vi "_f_BronkhorstModule.vi"(5 "Enable(T)":bool=TRUE, 6 "Delay":dbl=0.05, 7 "Command":T2, 8 "error in (no error)":errorcluster, 9 "Value":dbl, 10 "Nodo":u8=3, 11 "VISA resource name":refnum<visa-resource-name>="COM1") -> (0 "error out":errorcluster, 1 "Reading":T3, 2 "Result":string, 3 "Value":string)   [LabVIEW 2013]
uses:
  _f_BronkhorstModuleControl.ctl
  SerialComm/_f_SerialComm_Hardware_Module Control.ctl
panel:
  out "commandType":T1(ring)
  in  "InitComms":bool
  out "ReadString":string
  out "SendString":string
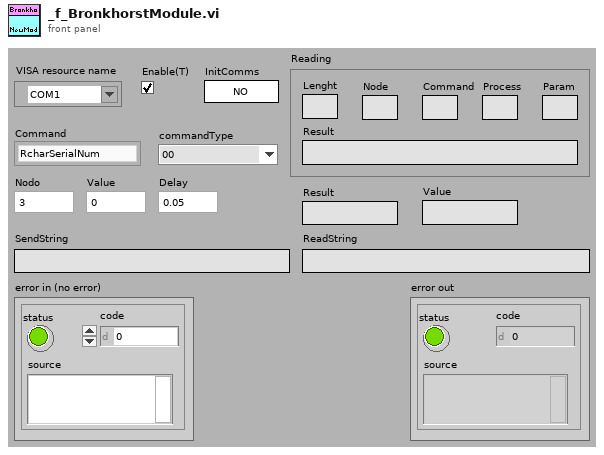
[diagram p1: front panel]
types:
  T1 = enum16{"00", "01", "02", "03", "04", "05", "06", "07", "08", "09"}
  T2 = typedef "_f_BronkhorstModuleControl.ctl" = enum16{"RcharSerialNum", "RcharIdnString", "WuintFluidNum", "RuintFluidNum", "RcharFluidName", "RuintSensorType", "RfloatCap0", "RfloatCap100", "RcharCapUnitStr", "W%Setpoint", "R%Setpoint", "R%Measure", "WfloatSetpoint", "RfloatSetpoint", "RfloatMeasure ", "RfloatDensity", "WuintControlMode", "WcharRESET", "RfloatCounter", "RcharCounterUnit", "WfloatCounterLimit", "RfloatCounterLimit", "WcharCounterMode", "RcharCounterMode", "WcharCounterSPMode", "RcharCounterSPMode", "WcharCounterNewSP", "RcharCounterNewSP"}
  T3 = cluster{"Lenght":string, "Node":string, "Process":string, "Param":string, "Command":string, "Result":string}
  T4 = typedef "_f_SerialComm_Hardware_Module Control.ctl" = enum16{"Initialize", "Write", "Bytes?", "Read", "Shutdown"}
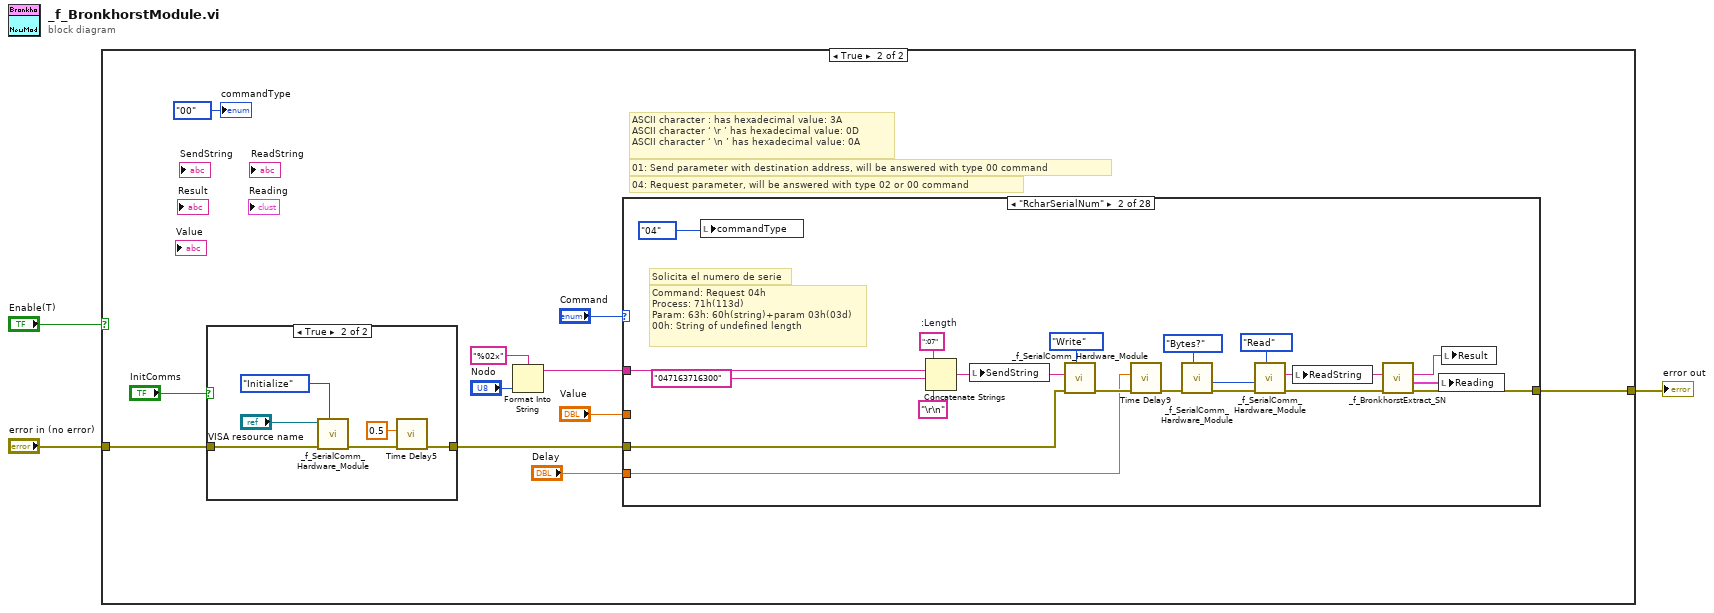
[diagram p0: block diagram]
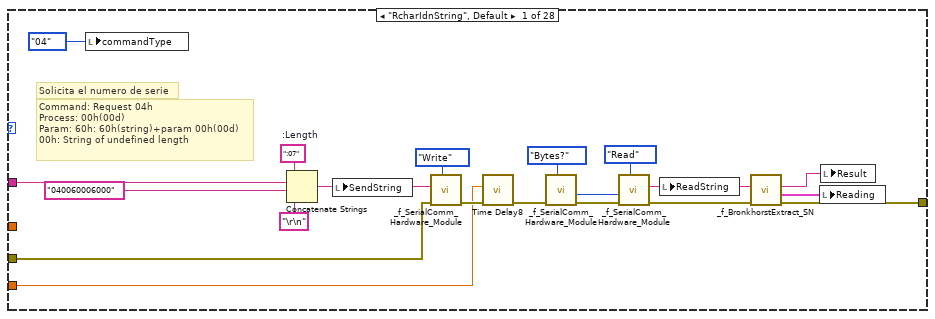
[diagram p4: hidden frame]
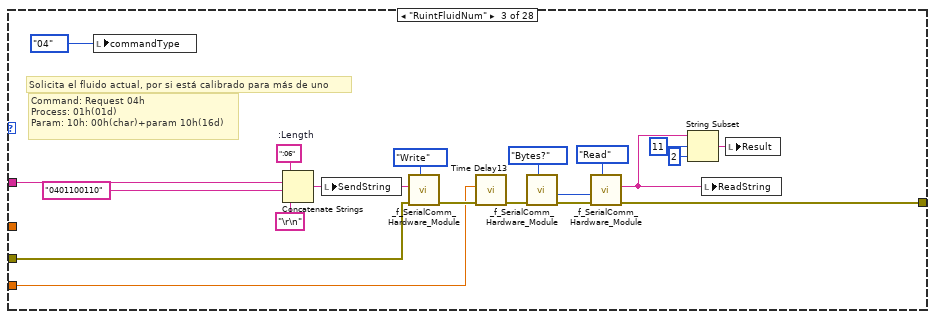
[diagram p5: hidden frame]
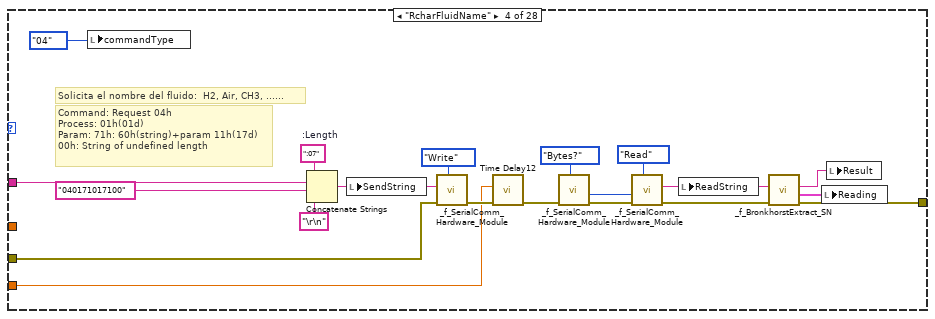
[diagram p6: hidden frame]
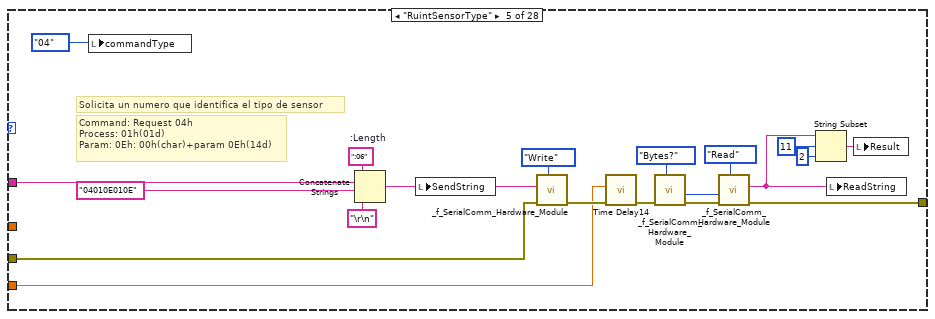
[diagram p7: hidden frame]
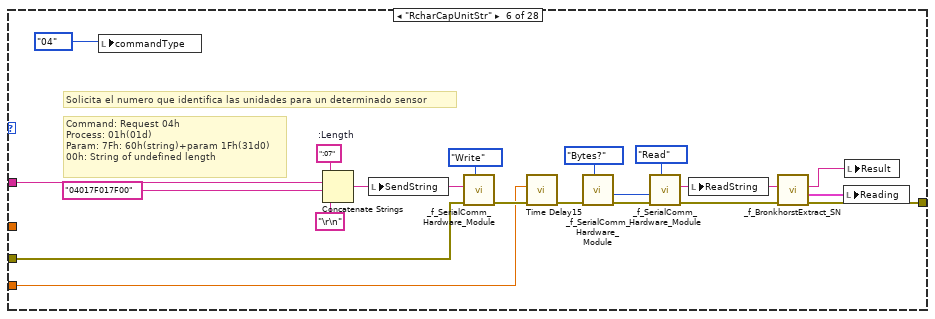
[diagram p8: hidden frame]
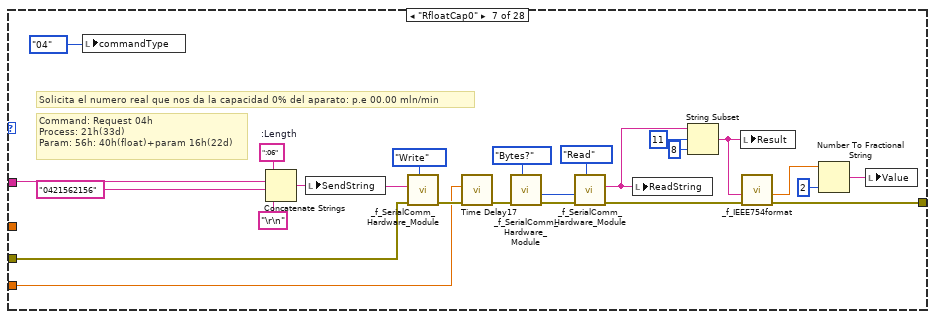
[diagram p9: hidden frame]
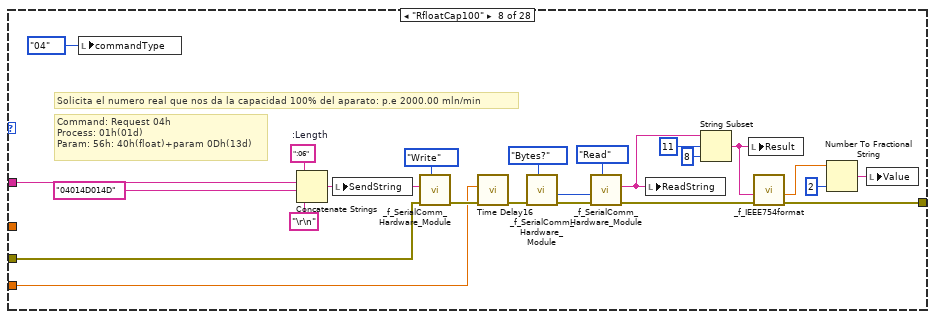
[diagram p10: hidden frame]
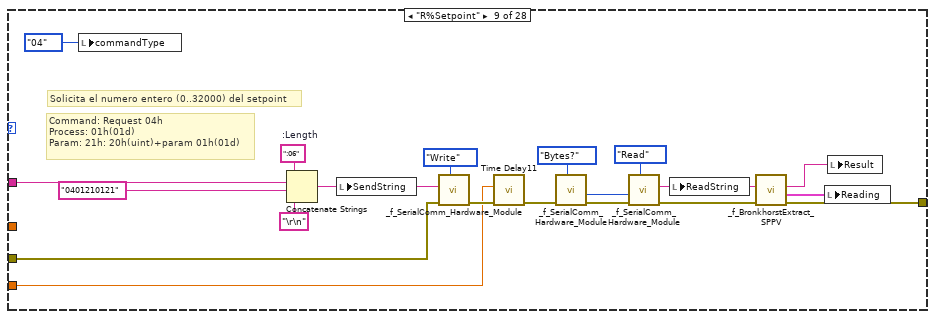
[diagram p11: hidden frame]
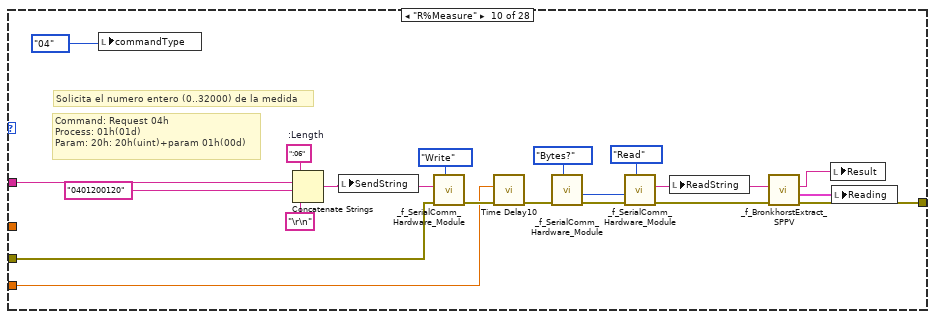
[diagram p12: hidden frame]
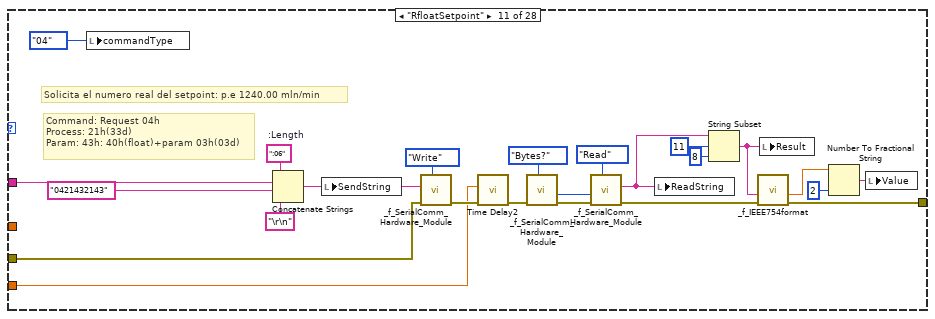
[diagram p13: hidden frame]
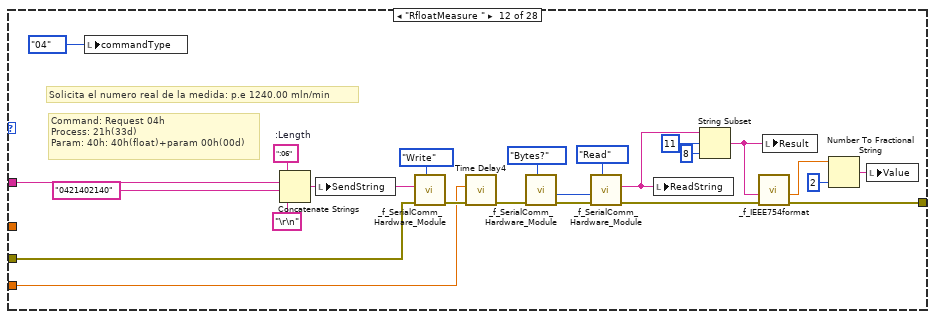
[diagram p14: hidden frame]
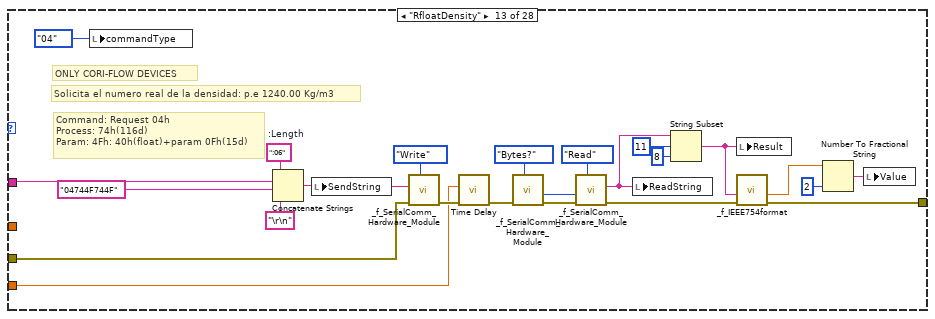
[diagram p15: hidden frame]
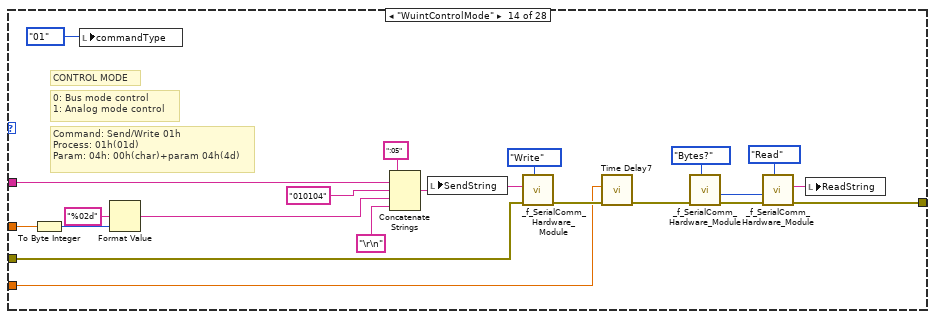
[diagram p16: hidden frame]
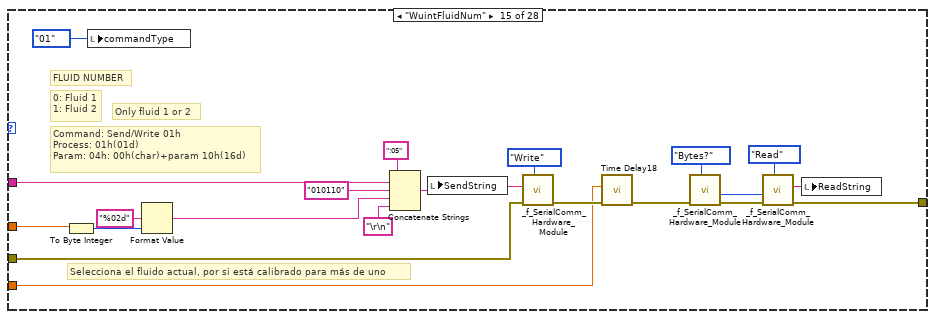
[diagram p17: hidden frame]
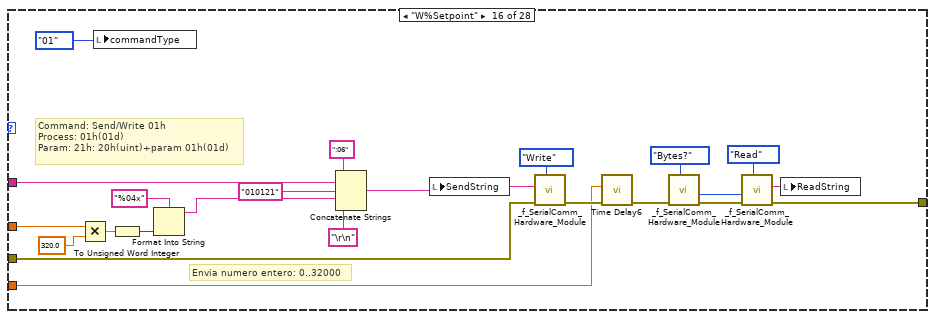
[diagram p18: hidden frame]
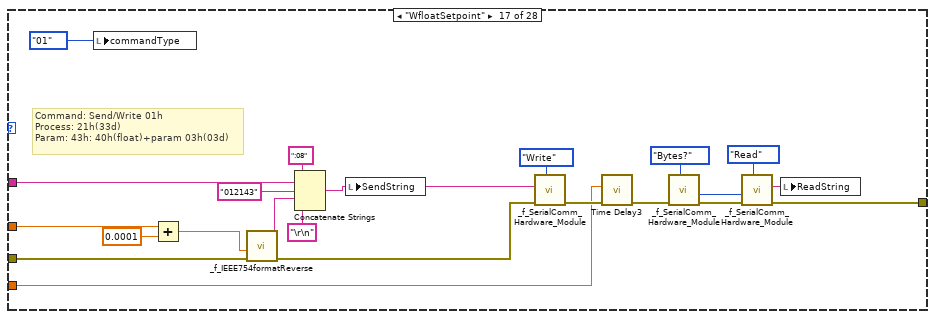
[diagram p19: hidden frame]
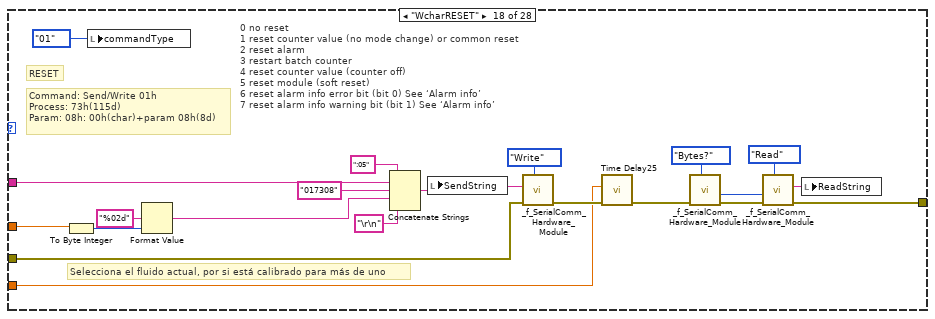
[diagram p20: hidden frame]
diagram:
  n1 = case shown="True" "Enable(T)" {
    tunnel: "error in (no error)" -> [w4 w14]
    tunnel: [w4 w5] -> w2
    frame False {
    }
    frame True {
      # "ASCII character : has hexadecimal value: 3A\nASCII character ‘ \\r ’ has hexadecimal value: 0D\nASCII character ‘ \\n ’ has hexadecimal value: 0A"
      # "04: Request parameter, will be answered with type 02 or 00 command"
      # "01: Send parameter with destination address, will be answered with type 00 command"
      n2 = case shown="True" "InitComms" {
        tunnel: w14 -> [w16 w21]
        tunnel: [w16 w18] -> w7
        frame False {
        }
        frame True {
          n3 = call "_f_SerialComm_Hardware_Module.vi"("Command"=_f_SerialComm_Hardware_Module_Control."Initialize", "error in (no error)"=w21, "VISA resource name"="VISA resource name") -> ("error out"=w19:errorcluster)  [unwired: 6 in, 2 out]
          n4 = call "Time Delay5"("error in (no error)"=w19, "Delay Time (s)"=0.5) -> ("error out"=w18:errorcluster)  [unwired: 9 in]
        }
      }
      n5 = Format Into String(format string="%02x", "Nodo") -> (resulting string=w10:string)  [unwired: 2 in, 1 out]
      n6 = case shown="\"RcharSerialNum\"" "Command" {
        tunnel: w10 -> [w24 w61 w64 w84 w104 w130 w144 w169 w193 w212 w233 w266 w281 w322 w343 w366 w388 w409 w413 w442 w473 w477 w518 w521 w559 w562 w602 w606]
        tunnel: w7 -> [w41 w59 w81 w101 w121 w141 w165 w189 w209 w229 w253 w277 w301 w320 w341 w363 w373 w407 w433 w453 w458 w497 w516 w538 w557 w579 w599 w622]
        tunnel: [w33 w51 w72 w93 w112 w124 w152 w173 w201 w221 w240 w259 w288 w311 w332 w354 w377 w398 w420 w436 w462 w484 w507 w529 w548 w570 w590 w614] -> w5
        tunnel: "Value" -> [_ _ _ _ _ _ _ _ _ _ _ _ _ w306 w326 w348 w374 w392 _ _ w459 _ w502 _ w543 _ w584 _]
        tunnel: "Delay" -> [w29 w46 w69 w89 w109 w134 w155 w179 w197 w217 w243 w270 w291 w310 w331 w346 w375 w397 w423 w446 w460 w487 w506 w526 w547 w567 w582 w610]
        frame "RcharIdnString", Default {
          w28 = ":07"  # :Length
          # "Command: Request 04h\nProcess: 00h(00d)\nParam: 60h: 60h(string)+param 00h(00d)\n00h: String of undefined length"
          # "Solicita el numero de serie"
          n7 = local write "commandType"(T1."04" ("commandType")) -> ()
          n8 = Concatenate Strings(w28, w24, "040060006000" ("string"), "\r\n" ("string")) -> (w25:string)
          n9 = local write "SendString"(w25) -> ()
          n10 = call "_f_SerialComm_Hardware_Module.vi"("Command"=_f_SerialComm_Hardware_Module_Control."Write", "error in (no error)"=w41, "Write string"=w25) -> ("error out"=w38:errorcluster)  [unwired: 6 in, 2 out]
          n11 = call "Time Delay8"("error in (no error)"=w38, "Delay Time (s)"=w29) -> ("error out"=w37:errorcluster)  [unwired: 9 in]
          n12 = call "_f_SerialComm_Hardware_Module.vi"("Command"=_f_SerialComm_Hardware_Module_Control."Bytes?", "error in (no error)"=w37) -> ("error out"=w36:errorcluster, "Bytes?"=w35:u32)  [unwired: 7 in, 1 out]
          n13 = call "_f_SerialComm_Hardware_Module.vi"("Command"=_f_SerialComm_Hardware_Module_Control."Read", "error in (no error)"=w36, "Bytes to read"=w35) -> ("error out"=w34:errorcluster, "Read string"=w32:string)  [unwired: 6 in, 1 out]
          n14 = local write "ReadString"(w32) -> ()
          n15 = call "_f_BronkhorstExtract_SN.vi"("error in (no error)"=w34, "Read String"=w32) -> ("error out"=w33:errorcluster, "Reading"=w31:T3, "Result"=w30:string)  [unwired: 7 in]
          n16 = local write "Reading"(w31) -> ()
          n17 = local write "Result"(w30) -> ()
        }
        frame "RcharSerialNum" {
          w62 = ":07"  # :Length
          # "Command: Request 04h\nProcess: 71h(113d)\nParam: 63h: 60h(string)+param 03h(03d)\n00h: String of undefined length"
          # "Solicita el numero de serie"
          n18 = local write "commandType"(T1."04" ("commandType")) -> ()
          n19 = Concatenate Strings(w62, w61, "047163716300" ("string"), "\r\n" ("string")) -> (w50:string)
          n20 = local write "SendString"(w50) -> ()
          n21 = call "_f_SerialComm_Hardware_Module.vi"("Command"=_f_SerialComm_Hardware_Module_Control."Write", "error in (no error)"=w59, "Write string"=w50) -> ("error out"=w56:errorcluster)  [unwired: 6 in, 2 out]
          n22 = call "Time Delay9"("error in (no error)"=w56, "Delay Time (s)"=w46) -> ("error out"=w55:errorcluster)  [unwired: 9 in]
          n23 = call "_f_SerialComm_Hardware_Module.vi"("Command"=_f_SerialComm_Hardware_Module_Control."Bytes?", "error in (no error)"=w55) -> ("error out"=w54:errorcluster, "Bytes?"=w53:u32)  [unwired: 7 in, 1 out]
          n24 = call "_f_SerialComm_Hardware_Module.vi"("Command"=_f_SerialComm_Hardware_Module_Control."Read", "error in (no error)"=w54, "Bytes to read"=w53) -> ("error out"=w52:errorcluster, "Read string"=w49:string)  [unwired: 6 in, 1 out]
          n25 = local write "ReadString"(w49) -> ()
          n26 = call "_f_BronkhorstExtract_SN.vi"("error in (no error)"=w52, "Read String"=w49) -> ("error out"=w51:errorcluster, "Reading"=w48:T3, "Result"=w47:string)  [unwired: 7 in]
          n27 = local write "Reading"(w48) -> ()
          n28 = local write "Result"(w47) -> ()
        }
        frame "RuintFluidNum" {
          w68 = ":06"  # :Length
          # "Command: Request 04h\nProcess: 01h(01d)\nParam: 10h: 00h(char)+param 10h(16d)"
          # "Solicita el fluido actual, por si está calibrado para más de uno"
          n29 = local write "commandType"(T1."04" ("commandType")) -> ()
          n30 = Concatenate Strings(w68, w64, "0401100110" ("string"), "\r\n" ("string")) -> (w65:string)
          n31 = local write "SendString"(w65) -> ()
          n32 = call "_f_SerialComm_Hardware_Module.vi"("Command"=_f_SerialComm_Hardware_Module_Control."Write", "error in (no error)"=w81, "Write string"=w65) -> ("error out"=w78:errorcluster)  [unwired: 6 in, 2 out]
          n33 = call "Time Delay13"("error in (no error)"=w78, "Delay Time (s)"=w69) -> ("error out"=w77:errorcluster)  [unwired: 9 in]
          n34 = call "_f_SerialComm_Hardware_Module.vi"("Command"=_f_SerialComm_Hardware_Module_Control."Bytes?", "error in (no error)"=w77) -> ("error out"=w76:errorcluster, "Bytes?"=w75:u32)  [unwired: 7 in, 1 out]
          n35 = call "_f_SerialComm_Hardware_Module.vi"("Command"=_f_SerialComm_Hardware_Module_Control."Read", "error in (no error)"=w76, "Bytes to read"=w75) -> ("error out"=w72:errorcluster, "Read string"=w73:string)  [unwired: 6 in, 1 out]
          n36 = String Subset(string=w73, offset (0)=11, length (rest)=2 ("length (rest)")) -> (substring=w70:string)
          n37 = local write "ReadString"(w73) -> ()
          n38 = local write "Result"(w70) -> ()
        }
        frame "RcharFluidName" {
          w88 = ":07"  # :Length
          # "Command: Request 04h\nProcess: 01h(01d)\nParam: 71h: 60h(string)+param 11h(17d)\n00h: String of undefined length"
          # "Solicita el nombre del fluido:  H2, Air, CH3, ......"
          n39 = local write "commandType"(T1."04" ("commandType")) -> ()
          n40 = Concatenate Strings(w88, w84, "040171017100" ("string"), "\r\n" ("string")) -> (w85:string)
          n41 = local write "SendString"(w85) -> ()
          n42 = call "_f_SerialComm_Hardware_Module.vi"("Command"=_f_SerialComm_Hardware_Module_Control."Write", "error in (no error)"=w101, "Write string"=w85) -> ("error out"=w98:errorcluster)  [unwired: 6 in, 2 out]
          n43 = call "Time Delay12"("error in (no error)"=w98, "Delay Time (s)"=w89) -> ("error out"=w97:errorcluster)  [unwired: 9 in]
          n44 = call "_f_SerialComm_Hardware_Module.vi"("Command"=_f_SerialComm_Hardware_Module_Control."Bytes?", "error in (no error)"=w97) -> ("error out"=w96:errorcluster, "Bytes?"=w95:u32)  [unwired: 7 in, 1 out]
          n45 = call "_f_SerialComm_Hardware_Module.vi"("Command"=_f_SerialComm_Hardware_Module_Control."Read", "error in (no error)"=w96, "Bytes to read"=w95) -> ("error out"=w94:errorcluster, "Read string"=w92:string)  [unwired: 6 in, 1 out]
          n46 = local write "ReadString"(w92) -> ()
          n47 = call "_f_BronkhorstExtract_SN.vi"("error in (no error)"=w94, "Read String"=w92) -> ("error out"=w93:errorcluster, "Reading"=w91:T3, "Result"=w90:string)  [unwired: 7 in]
          n48 = local write "Reading"(w91) -> ()
          n49 = local write "Result"(w90) -> ()
        }
        frame "RuintSensorType" {
          w108 = ":06"  # :Length
          # "Command: Request 04h\nProcess: 01h(01d)\nParam: 0Eh: 00h(char)+param 0Eh(14d)"
          # "Solicita un numero que identifica el tipo de sensor"
          n50 = local write "commandType"(T1."04" ("commandType")) -> ()
          n51 = Concatenate Strings(w108, w104, "04010E010E" ("string"), "\r\n" ("string")) -> (w105:string)
          n52 = local write "SendString"(w105) -> ()
          n53 = call "_f_SerialComm_Hardware_Module.vi"("Command"=_f_SerialComm_Hardware_Module_Control."Write", "error in (no error)"=w121, "Write string"=w105) -> ("error out"=w118:errorcluster)  [unwired: 6 in, 2 out]
          n54 = call "Time Delay14"("error in (no error)"=w118, "Delay Time (s)"=w109) -> ("error out"=w117:errorcluster)  [unwired: 9 in]
          n55 = call "_f_SerialComm_Hardware_Module.vi"("Command"=_f_SerialComm_Hardware_Module_Control."Bytes?", "error in (no error)"=w117) -> ("error out"=w116:errorcluster, "Bytes?"=w115:u32)  [unwired: 7 in, 1 out]
          n56 = call "_f_SerialComm_Hardware_Module.vi"("Command"=_f_SerialComm_Hardware_Module_Control."Read", "error in (no error)"=w116, "Bytes to read"=w115) -> ("error out"=w112:errorcluster, "Read string"=w113:string)  [unwired: 6 in, 1 out]
          n57 = String Subset(string=w113, offset (0)=11, length (rest)=2 ("length (rest)")) -> (substring=w110:string)
          n58 = local write "ReadString"(w113) -> ()
          n59 = local write "Result"(w110) -> ()
        }
        frame "RcharCapUnitStr" {
          w133 = ":07"  # :Length
          # "Command: Request 04h\nProcess: 01h(01d)\nParam: 7Fh: 60h(string)+param 1Fh(31d0)\n00h: String of undefined length"
          # "Solicita el numero que identifica las unidades para un determinado sensor"
          n60 = local write "commandType"(T1."04" ("commandType")) -> ()
          n61 = Concatenate Strings(w133, w130, "04017F017F00" ("string"), "\r\n" ("string")) -> (w129:string)
          n62 = local write "SendString"(w129) -> ()
          n63 = call "_f_SerialComm_Hardware_Module.vi"("Command"=_f_SerialComm_Hardware_Module_Control."Write", "error in (no error)"=w141, "Write string"=w129) -> ("error out"=w138:errorcluster)  [unwired: 6 in, 2 out]
          n64 = call "Time Delay15"("error in (no error)"=w138, "Delay Time (s)"=w134) -> ("error out"=w137:errorcluster)  [unwired: 9 in]
          n65 = call "_f_SerialComm_Hardware_Module.vi"("Command"=_f_SerialComm_Hardware_Module_Control."Bytes?", "error in (no error)"=w137) -> ("error out"=w136:errorcluster, "Bytes?"=w135:u32)  [unwired: 7 in, 1 out]
          n66 = call "_f_SerialComm_Hardware_Module.vi"("Command"=_f_SerialComm_Hardware_Module_Control."Read", "error in (no error)"=w136, "Bytes to read"=w135) -> ("error out"=w125:errorcluster, "Read string"=w128:string)  [unwired: 6 in, 1 out]
          n67 = local write "ReadString"(w128) -> ()
          n68 = call "_f_BronkhorstExtract_SN.vi"("error in (no error)"=w125, "Read String"=w128) -> ("error out"=w124:errorcluster, "Reading"=w126:T3, "Result"=w127:string)  [unwired: 7 in]
          n69 = local write "Reading"(w126) -> ()
          n70 = local write "Result"(w127) -> ()
        }
        frame "RfloatCap0" {
          w148 = ":06"  # :Length
          # "Command: Request 04h\nProcess: 21h(33d)\nParam: 56h: 40h(float)+param 16h(22d)"
          # "Solicita el numero real que nos da la capacidad 0% del aparato: p.e 00.00 mln/min"
          n71 = local write "commandType"(T1."04" ("commandType")) -> ()
          n72 = Concatenate Strings(w148, w144, "0421562156" ("string"), "\r\n" ("string")) -> (w145:string)
          n73 = local write "SendString"(w145) -> ()
          n74 = call "_f_SerialComm_Hardware_Module.vi"("Command"=_f_SerialComm_Hardware_Module_Control."Write", "error in (no error)"=w165, "Write string"=w145) -> ("error out"=w162:errorcluster)  [unwired: 6 in, 2 out]
          n75 = call "Time Delay17"("error in (no error)"=w162, "Delay Time (s)"=w155) -> ("error out"=w161:errorcluster)  [unwired: 9 in]
          n76 = call "_f_SerialComm_Hardware_Module.vi"("Command"=_f_SerialComm_Hardware_Module_Control."Bytes?", "error in (no error)"=w161) -> ("error out"=w160:errorcluster, "Bytes?"=w159:u32)  [unwired: 7 in, 1 out]
          n77 = call "_f_SerialComm_Hardware_Module.vi"("Command"=_f_SerialComm_Hardware_Module_Control."Read", "error in (no error)"=w160, "Bytes to read"=w159) -> ("error out"=w153:errorcluster, "Read string"=w157:string)  [unwired: 6 in, 1 out]
          n78 = local write "ReadString"(w157) -> ()
          n79 = String Subset(string=w157, offset (0)=11, length (rest)=8 ("length (rest)")) -> (substring=w154:string)
          n80 = local write "Result"(w154) -> ()
          n81 = call "_f_IEEE754format.vi"("error in (no error)"=w153, "String"=w154) -> ("error out"=w152:errorcluster, "Number"=w149:sgl)  [unwired: 8 in]
          n82 = Number To Fractional String(number=w149, precision (6)=i16 2) -> (F-format string=w150:string)  [unwired: 2 in]
          n83 = local write "Value"(w150) -> ()
        }
        frame "RfloatCap100" {
          w172 = ":06"  # :Length
          # "Command: Request 04h\nProcess: 01h(01d)\nParam: 56h: 40h(float)+param 0Dh(13d)"
          # "Solicita el numero real que nos da la capacidad 100% del aparato: p.e 2000.00 mln/min"
          n84 = local write "commandType"(T1."04" ("commandType")) -> ()
          n85 = Concatenate Strings(w172, w169, "04014D014D" ("string"), "\r\n" ("string")) -> (w168:string)
          n86 = local write "SendString"(w168) -> ()
          n87 = call "_f_SerialComm_Hardware_Module.vi"("Command"=_f_SerialComm_Hardware_Module_Control."Write", "error in (no error)"=w189, "Write string"=w168) -> ("error out"=w186:errorcluster)  [unwired: 6 in, 2 out]
          n88 = call "Time Delay16"("error in (no error)"=w186, "Delay Time (s)"=w179) -> ("error out"=w185:errorcluster)  [unwired: 9 in]
          n89 = call "_f_SerialComm_Hardware_Module.vi"("Command"=_f_SerialComm_Hardware_Module_Control."Bytes?", "error in (no error)"=w185) -> ("error out"=w184:errorcluster, "Bytes?"=w183:u32)  [unwired: 7 in, 1 out]
          n90 = call "_f_SerialComm_Hardware_Module.vi"("Command"=_f_SerialComm_Hardware_Module_Control."Read", "error in (no error)"=w184, "Bytes to read"=w183) -> ("error out"=w174:errorcluster, "Read string"=w181:string)  [unwired: 6 in, 1 out]
          n91 = local write "ReadString"(w181) -> ()
          n92 = String Subset(string=w181, offset (0)=11, length (rest)=8 ("length (rest)")) -> (substring=w176:string)
          n93 = local write "Result"(w176) -> ()
          n94 = call "_f_IEEE754format.vi"("error in (no error)"=w174, "String"=w176) -> ("error out"=w173:errorcluster, "Number"=w175:sgl)  [unwired: 8 in]
          n95 = Number To Fractional String(number=w175, precision (6)=i16 2) -> (F-format string=w177:string)  [unwired: 2 in]
          n96 = local write "Value"(w177) -> ()
        }
        frame "R%Setpoint" {
          w196 = ":06"  # :Length
          # "Command: Request 04h\nProcess: 01h(01d)\nParam: 21h: 20h(uint)+param 01h(01d)"
          # "Solicita el numero entero (0..32000) del setpoint"
          n97 = local write "commandType"(T1."04" ("commandType")) -> ()
          n98 = Concatenate Strings(w196, w193, "0401210121" ("string"), "\r\n" ("string")) -> (w192:string)
          n99 = local write "SendString"(w192) -> ()
          n100 = call "_f_SerialComm_Hardware_Module.vi"("Command"=_f_SerialComm_Hardware_Module_Control."Write", "error in (no error)"=w209, "Write string"=w192) -> ("error out"=w206:errorcluster)  [unwired: 6 in, 2 out]
          n101 = call "Time Delay11"("error in (no error)"=w206, "Delay Time (s)"=w197) -> ("error out"=w205:errorcluster)  [unwired: 9 in]
          n102 = call "_f_SerialComm_Hardware_Module.vi"("Command"=_f_SerialComm_Hardware_Module_Control."Bytes?", "error in (no error)"=w205) -> ("error out"=w204:errorcluster, "Bytes?"=w203:u32)  [unwired: 7 in, 1 out]
          n103 = call "_f_SerialComm_Hardware_Module.vi"("Command"=_f_SerialComm_Hardware_Module_Control."Read", "error in (no error)"=w204, "Bytes to read"=w203) -> ("error out"=w202:errorcluster, "Read string"=w200:string)  [unwired: 6 in, 1 out]
          n104 = local write "ReadString"(w200) -> ()
          n105 = call "_f_BronkhorstExtract_SPPV.vi"("error in (no error)"=w202, "Read String"=w200) -> ("error out"=w201:errorcluster, "Reading"=w199:T3, "Setpoint"=w198:string)  [unwired: 7 in]
          n106 = local write "Reading"(w199) -> ()
          n107 = local write "Result"(w198) -> ()
        }
        frame "R%Measure" {
          w216 = ":06"  # :Length
          # "Command: Request 04h\nProcess: 01h(01d)\nParam: 20h: 20h(uint)+param 01h(00d)"
          # "Solicita el numero entero (0..32000) de la medida"
          n108 = local write "commandType"(T1."04" ("commandType")) -> ()
          n109 = Concatenate Strings(w216, w212, "0401200120" ("string"), "\r\n" ("string")) -> (w213:string)
          n110 = local write "SendString"(w213) -> ()
          n111 = call "_f_SerialComm_Hardware_Module.vi"("Command"=_f_SerialComm_Hardware_Module_Control."Write", "error in (no error)"=w229, "Write string"=w213) -> ("error out"=w226:errorcluster)  [unwired: 6 in, 2 out]
          n112 = call "Time Delay10"("error in (no error)"=w226, "Delay Time (s)"=w217) -> ("error out"=w225:errorcluster)  [unwired: 9 in]
          n113 = call "_f_SerialComm_Hardware_Module.vi"("Command"=_f_SerialComm_Hardware_Module_Control."Bytes?", "error in (no error)"=w225) -> ("error out"=w224:errorcluster, "Bytes?"=w223:u32)  [unwired: 7 in, 1 out]
          n114 = call "_f_SerialComm_Hardware_Module.vi"("Command"=_f_SerialComm_Hardware_Module_Control."Read", "error in (no error)"=w224, "Bytes to read"=w223) -> ("error out"=w222:errorcluster, "Read string"=w219:string)  [unwired: 6 in, 1 out]
          n115 = local write "ReadString"(w219) -> ()
          n116 = call "_f_BronkhorstExtract_SPPV.vi"("error in (no error)"=w222, "Read String"=w219) -> ("error out"=w221:errorcluster, "Reading"=w220:T3, "Setpoint"=w218:string)  [unwired: 7 in]
          n117 = local write "Result"(w218) -> ()
          n118 = local write "Reading"(w220) -> ()
        }
        frame "RfloatSetpoint" {
          w236 = ":06"  # :Length
          # "Command: Request 04h\nProcess: 21h(33d)\nParam: 43h: 40h(float)+param 03h(03d)"
          # "Solicita el numero real del setpoint: p.e 1240.00 mln/min"
          n119 = local write "commandType"(T1."04" ("commandType")) -> ()
          n120 = Concatenate Strings(w236, w233, "0421432143" ("string"), "\r\n" ("string")) -> (w232:string)
          n121 = local write "SendString"(w232) -> ()
          n122 = call "_f_SerialComm_Hardware_Module.vi"("Command"=_f_SerialComm_Hardware_Module_Control."Write", "error in (no error)"=w253, "Write string"=w232) -> ("error out"=w250:errorcluster)  [unwired: 6 in, 2 out]
          n123 = call "Time Delay2"("error in (no error)"=w250, "Delay Time (s)"=w243) -> ("error out"=w249:errorcluster)  [unwired: 9 in]
          n124 = call "_f_SerialComm_Hardware_Module.vi"("Command"=_f_SerialComm_Hardware_Module_Control."Bytes?", "error in (no error)"=w249) -> ("error out"=w248:errorcluster, "Bytes?"=w247:u32)  [unwired: 7 in, 1 out]
          n125 = call "_f_SerialComm_Hardware_Module.vi"("Command"=_f_SerialComm_Hardware_Module_Control."Read", "error in (no error)"=w248, "Bytes to read"=w247) -> ("error out"=w241:errorcluster, "Read string"=w245:string)  [unwired: 6 in, 1 out]
          n126 = local write "ReadString"(w245) -> ()
          n127 = String Subset(string=w245, offset (0)=11, length (rest)=8 ("length (rest)")) -> (substring=w242:string)
          n128 = call "_f_IEEE754format.vi"("error in (no error)"=w241, "String"=w242) -> ("error out"=w240:errorcluster, "Number"=w238:sgl)  [unwired: 8 in]
          n129 = local write "Result"(w242) -> ()
          n130 = Number To Fractional String(number=w238, precision (6)=i16 2) -> (F-format string=w237:string)  [unwired: 2 in]
          n131 = local write "Value"(w237) -> ()
        }
        frame "RfloatMeasure " {
          w269 = ":06"  # :Length
          # "Command: Request 04h\nProcess: 21h(33d)\nParam: 40h: 40h(float)+param 00h(00d)"
          # "Solicita el numero real de la medida: p.e 1240.00 mln/min"
          n132 = local write "commandType"(T1."04" ("commandType")) -> ()
          n133 = Concatenate Strings(w269, w266, "0421402140" ("string"), "\r\n" ("string")) -> (w265:string)
          n134 = local write "SendString"(w265) -> ()
          n135 = call "_f_SerialComm_Hardware_Module.vi"("Command"=_f_SerialComm_Hardware_Module_Control."Write", "error in (no error)"=w277, "Write string"=w265) -> ("error out"=w274:errorcluster)  [unwired: 6 in, 2 out]
          n136 = call "Time Delay4"("error in (no error)"=w274, "Delay Time (s)"=w270) -> ("error out"=w273:errorcluster)  [unwired: 9 in]
          n137 = call "_f_SerialComm_Hardware_Module.vi"("Command"=_f_SerialComm_Hardware_Module_Control."Bytes?", "error in (no error)"=w273) -> ("error out"=w272:errorcluster, "Bytes?"=w271:u32)  [unwired: 7 in, 1 out]
          n138 = call "_f_SerialComm_Hardware_Module.vi"("Command"=_f_SerialComm_Hardware_Module_Control."Read", "error in (no error)"=w272, "Bytes to read"=w271) -> ("error out"=w260:errorcluster, "Read string"=w258:string)  [unwired: 6 in, 1 out]
          n139 = local write "ReadString"(w258) -> ()
          n140 = String Subset(string=w258, offset (0)=11, length (rest)=8 ("length (rest)")) -> (substring=w257:string)
          n141 = call "_f_IEEE754format.vi"("error in (no error)"=w260, "String"=w257) -> ("error out"=w259:errorcluster, "Number"=w256:sgl)  [unwired: 8 in]
          n142 = local write "Result"(w257) -> ()
          n143 = Number To Fractional String(number=w256, precision (6)=i16 2) -> (F-format string=w261:string)  [unwired: 2 in]
          n144 = local write "Value"(w261) -> ()
        }
        frame "RfloatDensity" {
          w284 = ":06"  # :Length
          # "ONLY CORI-FLOW DEVICES"
          # "Command: Request 04h\nProcess: 74h(116d)\nParam: 4Fh: 40h(float)+param 0Fh(15d)"
          # "Solicita el numero real de la densidad: p.e 1240.00 Kg/m3"
          n145 = local write "commandType"(T1."04" ("commandType")) -> ()
          n146 = Concatenate Strings(w284, w281, "04744F744F" ("string"), "\r\n" ("string")) -> (w280:string)
          n147 = local write "SendString"(w280) -> ()
          n148 = call "_f_SerialComm_Hardware_Module.vi"("Command"=_f_SerialComm_Hardware_Module_Control."Write", "error in (no error)"=w301, "Write string"=w280) -> ("error out"=w298:errorcluster)  [unwired: 6 in, 2 out]
          n149 = call "Time Delay"("error in (no error)"=w298, "Delay Time (s)"=w291) -> ("error out"=w297:errorcluster)  [unwired: 9 in]
          n150 = call "_f_SerialComm_Hardware_Module.vi"("Command"=_f_SerialComm_Hardware_Module_Control."Bytes?", "error in (no error)"=w297) -> ("error out"=w296:errorcluster, "Bytes?"=w295:u32)  [unwired: 7 in, 1 out]
          n151 = call "_f_SerialComm_Hardware_Module.vi"("Command"=_f_SerialComm_Hardware_Module_Control."Read", "error in (no error)"=w296, "Bytes to read"=w295) -> ("error out"=w289:errorcluster, "Read string"=w293:string)  [unwired: 6 in, 1 out]
          n152 = local write "ReadString"(w293) -> ()
          n153 = String Subset(string=w293, offset (0)=11, length (rest)=8 ("length (rest)")) -> (substring=w290:string)
          n154 = local write "Result"(w290) -> ()
          n155 = call "_f_IEEE754format.vi"("error in (no error)"=w289, "String"=w290) -> ("error out"=w288:errorcluster, "Number"=w286:sgl)  [unwired: 8 in]
          n156 = Number To Fractional String(number=w286, precision (6)=i16 2) -> (F-format string=w285:string)  [unwired: 2 in]
          n157 = local write "Value"(w285) -> ()
        }
        frame "WuintControlMode" {
          # "CONTROL MODE"
          # "Command: Send/Write 01h\nProcess: 01h(01d)\nParam: 04h: 00h(char)+param 04h(4d)"
          # "0: Bus mode control\n1: Analog mode control"
          n158 = To Byte Integer(number=w306) -> (8bit integer=w308:i8)
          n159 = local write "commandType"(T1."01" ("commandType")) -> ()
          n160 = Format Value(format string="%02d", value (0)=w308) -> (output string=w303:string)  [unwired: 1 in]
          n161 = Concatenate Strings(":05" ("string"), w322, "010104", w303, "\r\n" ("string")) -> (w313:string)
          n162 = local write "SendString"(w313) -> ()
          n163 = call "_f_SerialComm_Hardware_Module.vi"("Command"=_f_SerialComm_Hardware_Module_Control."Write", "error in (no error)"=w320, "Write string"=w313) -> ("error out"=w317:errorcluster)  [unwired: 6 in, 2 out]
          n164 = call "Time Delay7"("error in (no error)"=w317, "Delay Time (s)"=w310) -> ("error out"=w316:errorcluster)  [unwired: 9 in]
          n165 = call "_f_SerialComm_Hardware_Module.vi"("Command"=_f_SerialComm_Hardware_Module_Control."Bytes?", "error in (no error)"=w316) -> ("error out"=w315:errorcluster, "Bytes?"=w314:u32)  [unwired: 7 in, 1 out]
          n166 = call "_f_SerialComm_Hardware_Module.vi"("Command"=_f_SerialComm_Hardware_Module_Control."Read", "error in (no error)"=w315, "Bytes to read"=w314) -> ("error out"=w311:errorcluster, "Read string"=w312:string)  [unwired: 6 in, 1 out]
          n167 = local write "ReadString"(w312) -> ()
        }
        frame "WuintFluidNum" {
          # "Selecciona el fluido actual, por si está calibrado para más de uno"
          # "Only fluid 1 or 2"
          # "FLUID NUMBER"
          # "Command: Send/Write 01h\nProcess: 01h(01d)\nParam: 04h: 00h(char)+param 10h(16d)"
          # "0: Fluid 1\n1: Fluid 2"
          n168 = To Byte Integer(number=w326) -> (8bit integer=w328:i8)
          n169 = local write "commandType"(T1."01" ("commandType")) -> ()
          n170 = Format Value(format string="%02d", value (0)=w328) -> (output string=w325:string)  [unwired: 1 in]
          n171 = Concatenate Strings(":05" ("string"), w343, "010110" ("Fluid 1"), w325, "\r\n" ("string")) -> (w334:string)
          n172 = local write "SendString"(w334) -> ()
          n173 = call "_f_SerialComm_Hardware_Module.vi"("Command"=_f_SerialComm_Hardware_Module_Control."Write", "error in (no error)"=w341, "Write string"=w334) -> ("error out"=w338:errorcluster)  [unwired: 6 in, 2 out]
          n174 = call "Time Delay18"("error in (no error)"=w338, "Delay Time (s)"=w331) -> ("error out"=w337:errorcluster)  [unwired: 9 in]
          n175 = call "_f_SerialComm_Hardware_Module.vi"("Command"=_f_SerialComm_Hardware_Module_Control."Bytes?", "error in (no error)"=w337) -> ("error out"=w336:errorcluster, "Bytes?"=w335:u32)  [unwired: 7 in, 1 out]
          n176 = call "_f_SerialComm_Hardware_Module.vi"("Command"=_f_SerialComm_Hardware_Module_Control."Read", "error in (no error)"=w336, "Bytes to read"=w335) -> ("error out"=w332:errorcluster, "Read string"=w333:string)  [unwired: 6 in, 1 out]
          n177 = local write "ReadString"(w333) -> ()
        }
        frame "W%Setpoint" {
          # "Command: Send/Write 01h\nProcess: 01h(01d)\nParam: 21h: 20h(uint)+param 01h(01d)"
          # "Envia numero entero: 0..32000"
          n178 = Multiply(x=w348, y=320.0) -> (x*y=w351:dbl)
          n179 = local write "commandType"(T1."01" ("commandType")) -> ()
          n180 = To Unsigned Word Integer(number=w351) -> (unsigned 16bit integer=w350:u16)
          n181 = Format Into String(format string="%04x", w350) -> (resulting string=w347:string)  [unwired: 2 in, 1 out]
          n182 = Concatenate Strings(":06" ("string"), w366, "010121" ("string"), w347, "\r\n" ("string")) -> (w356:string)
          n183 = local write "SendString"(w356) -> ()
          n184 = call "_f_SerialComm_Hardware_Module.vi"("Command"=_f_SerialComm_Hardware_Module_Control."Write", "error in (no error)"=w363, "Write string"=w356) -> ("error out"=w360:errorcluster)  [unwired: 6 in, 2 out]
          n185 = call "Time Delay6"("error in (no error)"=w360, "Delay Time (s)"=w346) -> ("error out"=w359:errorcluster)  [unwired: 9 in]
          n186 = call "_f_SerialComm_Hardware_Module.vi"("Command"=_f_SerialComm_Hardware_Module_Control."Bytes?", "error in (no error)"=w359) -> ("error out"=w358:errorcluster, "Bytes?"=w357:u32)  [unwired: 7 in, 1 out]
          n187 = call "_f_SerialComm_Hardware_Module.vi"("Command"=_f_SerialComm_Hardware_Module_Control."Read", "error in (no error)"=w358, "Bytes to read"=w357) -> ("error out"=w354:errorcluster, "Read string"=w355:string)  [unwired: 6 in, 1 out]
          n188 = local write "ReadString"(w355) -> ()
        }
        frame "WfloatSetpoint" {
          # "Command: Send/Write 01h\nProcess: 21h(33d)\nParam: 43h: 40h(float)+param 03h(03d)"
          n189 = local write "commandType"(T1."01" ("commandType")) -> ()
          n190 = Add(x=w374, y=0.0001) -> (x+y=w369:dbl)
          n191 = call "_f_IEEE754formatReverse.vi"("error in (no error)"=w373, "Number"=w369) -> ("error out"=w372:errorcluster, "String"=w371:string)  [unwired: 8 in]
          n192 = Concatenate Strings(":08" ("string"), w388, "012143" ("string"), w371, "\r\n" ("string")) -> (w379:string)
          n193 = local write "SendString"(w379) -> ()
          n194 = call "_f_SerialComm_Hardware_Module.vi"("Command"=_f_SerialComm_Hardware_Module_Control."Write", "error in (no error)"=w372, "Write string"=w379) -> ("error out"=w383:errorcluster)  [unwired: 6 in, 2 out]
          n195 = call "Time Delay3"("error in (no error)"=w383, "Delay Time (s)"=w375) -> ("error out"=w382:errorcluster)  [unwired: 9 in]
          n196 = call "_f_SerialComm_Hardware_Module.vi"("Command"=_f_SerialComm_Hardware_Module_Control."Bytes?", "error in (no error)"=w382) -> ("error out"=w381:errorcluster, "Bytes?"=w380:u32)  [unwired: 7 in, 1 out]
          n197 = call "_f_SerialComm_Hardware_Module.vi"("Command"=_f_SerialComm_Hardware_Module_Control."Read", "error in (no error)"=w381, "Bytes to read"=w380) -> ("error out"=w377:errorcluster, "Read string"=w378:string)  [unwired: 6 in, 1 out]
          n198 = local write "ReadString"(w378) -> ()
        }
        frame "WcharRESET" {
          # "0 no reset\n1 reset counter value (no mode change) or common reset\n2 reset alarm\n3 restart batch counter\n4 reset counter value (counter off)\n5 reset module (soft reset)\n6 reset alarm info error bit (bit 0) See ‘Alarm info’\n7 reset alarm info warning bit (bit 1) See ‘Alarm info’"
          # "Selecciona el fluido actual, por si está calibrado para más de uno"
          # "RESET"
          # "Command: Send/Write 01h\nProcess: 73h(115d)\nParam: 08h: 00h(char)+param 08h(8d)"
          n199 = To Byte Integer(number=w392) -> (8bit integer=w394:i8)
          n200 = local write "commandType"(T1."01" ("commandType")) -> ()
          n201 = Format Value(format string="%02d", value (0)=w394) -> (output string=w391:string)  [unwired: 1 in]
          n202 = Concatenate Strings(":05" ("string"), w409, "017308" ("Fluid 1"), w391, "\r\n" ("string")) -> (w400:string)
          n203 = local write "SendString"(w400) -> ()
          n204 = call "_f_SerialComm_Hardware_Module.vi"("Command"=_f_SerialComm_Hardware_Module_Control."Write", "error in (no error)"=w407, "Write string"=w400) -> ("error out"=w404:errorcluster)  [unwired: 6 in, 2 out]
          n205 = call "Time Delay25"("error in (no error)"=w404, "Delay Time (s)"=w397) -> ("error out"=w403:errorcluster)  [unwired: 9 in]
          n206 = call "_f_SerialComm_Hardware_Module.vi"("Command"=_f_SerialComm_Hardware_Module_Control."Bytes?", "error in (no error)"=w403) -> ("error out"=w402:errorcluster, "Bytes?"=w401:u32)  [unwired: 7 in, 1 out]
          n207 = call "_f_SerialComm_Hardware_Module.vi"("Command"=_f_SerialComm_Hardware_Module_Control."Read", "error in (no error)"=w402, "Bytes to read"=w401) -> ("error out"=w398:errorcluster, "Read string"=w399:string)  [unwired: 6 in, 1 out]
          n208 = local write "ReadString"(w399) -> ()
        }
        frame "RfloatCounter" {
          w416 = ":06"  # :Length
          # "Command: Request 04h\nProcess: 68h(104d)\nParam: 41h: 40h(float)+param 01h(1d)"
          # "Solicita el contador : p.e 1240.00 Kg"
          n209 = local write "commandType"(T1."04" ("commandType")) -> ()
          n210 = Concatenate Strings(w416, w413, "0468416841" ("string"), "\r\n" ("string")) -> (w412:string)
          n211 = local write "SendString"(w412) -> ()
          n212 = call "_f_SerialComm_Hardware_Module.vi"("Command"=_f_SerialComm_Hardware_Module_Control."Write", "error in (no error)"=w433, "Write string"=w412) -> ("error out"=w430:errorcluster)  [unwired: 6 in, 2 out]
          n213 = call "Time Delay19"("error in (no error)"=w430, "Delay Time (s)"=w423) -> ("error out"=w429:errorcluster)  [unwired: 9 in]
          n214 = call "_f_SerialComm_Hardware_Module.vi"("Command"=_f_SerialComm_Hardware_Module_Control."Bytes?", "error in (no error)"=w429) -> ("error out"=w428:errorcluster, "Bytes?"=w427:u32)  [unwired: 7 in, 1 out]
          n215 = call "_f_SerialComm_Hardware_Module.vi"("Command"=_f_SerialComm_Hardware_Module_Control."Read", "error in (no error)"=w428, "Bytes to read"=w427) -> ("error out"=w421:errorcluster, "Read string"=w425:string)  [unwired: 6 in, 1 out]
          n216 = local write "ReadString"(w425) -> ()
          n217 = String Subset(string=w425, offset (0)=11, length (rest)=8 ("length (rest)")) -> (substring=w422:string)
          n218 = local write "Result"(w422) -> ()
          n219 = call "_f_IEEE754format.vi"("error in (no error)"=w421, "String"=w422) -> ("error out"=w420:errorcluster, "Number"=w418:sgl)  [unwired: 8 in]
          n220 = Number To Fractional String(number=w418, precision (6)=i16 2) -> (F-format string=w417:string)  [unwired: 2 in]
          n221 = local write "Value"(w417) -> ()
        }
        frame "RcharCounterUnit" {
          w445 = ":07"  # :Length
          # "Command: Request 04h\nProcess: 68h(104d)\nParam: 67h: 60h(string)+param 07h(07d)\n00h: String of undefined length"
          # "Solicita el numero que identifica las unidades para un determinado sensor"
          n222 = local write "commandType"(T1."04" ("commandType")) -> ()
          n223 = Concatenate Strings(w445, w442, "046867686700" ("string"), "\r\n" ("string")) -> (w441:string)
          n224 = local write "SendString"(w441) -> ()
          n225 = call "_f_SerialComm_Hardware_Module.vi"("Command"=_f_SerialComm_Hardware_Module_Control."Write", "error in (no error)"=w453, "Write string"=w441) -> ("error out"=w450:errorcluster)  [unwired: 6 in, 2 out]
          n226 = call "Time Delay20"("error in (no error)"=w450, "Delay Time (s)"=w446) -> ("error out"=w449:errorcluster)  [unwired: 9 in]
          n227 = call "_f_SerialComm_Hardware_Module.vi"("Command"=_f_SerialComm_Hardware_Module_Control."Bytes?", "error in (no error)"=w449) -> ("error out"=w448:errorcluster, "Bytes?"=w447:u32)  [unwired: 7 in, 1 out]
          n228 = call "_f_SerialComm_Hardware_Module.vi"("Command"=_f_SerialComm_Hardware_Module_Control."Read", "error in (no error)"=w448, "Bytes to read"=w447) -> ("error out"=w437:errorcluster, "Read string"=w440:string)  [unwired: 6 in, 1 out]
          n229 = local write "ReadString"(w440) -> ()
          n230 = call "_f_BronkhorstExtract_SN.vi"("error in (no error)"=w437, "Read String"=w440) -> ("error out"=w436:errorcluster, "Reading"=w438:T3, "Result"=w439:string)  [unwired: 7 in]
          n231 = local write "Reading"(w438) -> ()
          n232 = local write "Result"(w439) -> ()
        }
        frame "WfloatCounterLimit" {
          # "Command: Send/Write 01h\nProcess: 68h(104d)\nParam: 43h: 40h(float)+param 03h(03d)"
          n233 = call "_f_IEEE754formatReverse.vi"("error in (no error)"=w458, "Number"=w459) -> ("error out"=w457:errorcluster, "String"=w456:string)  [unwired: 8 in]
          n234 = local write "commandType"(T1."01" ("commandType")) -> ()
          n235 = Concatenate Strings(":08" ("string"), w473, "016843" ("string"), w456, "\r\n" ("string")) -> (w464:string)
          n236 = local write "SendString"(w464) -> ()
          n237 = call "_f_SerialComm_Hardware_Module.vi"("Command"=_f_SerialComm_Hardware_Module_Control."Write", "error in (no error)"=w457, "Write string"=w464) -> ("error out"=w468:errorcluster)  [unwired: 6 in, 2 out]
          n238 = call "Time Delay22"("error in (no error)"=w468, "Delay Time (s)"=w460) -> ("error out"=w467:errorcluster)  [unwired: 9 in]
          n239 = call "_f_SerialComm_Hardware_Module.vi"("Command"=_f_SerialComm_Hardware_Module_Control."Bytes?", "error in (no error)"=w467) -> ("error out"=w466:errorcluster, "Bytes?"=w465:u32)  [unwired: 7 in, 1 out]
          n240 = call "_f_SerialComm_Hardware_Module.vi"("Command"=_f_SerialComm_Hardware_Module_Control."Read", "error in (no error)"=w466, "Bytes to read"=w465) -> ("error out"=w462:errorcluster, "Read string"=w463:string)  [unwired: 6 in, 1 out]
          n241 = local write "ReadString"(w463) -> ()
        }
        frame "RfloatCounterLimit" {
          w480 = ":06"  # :Length
          # "Command: Request 04h\nProcess: 68h(104d)\nParam: 41h: 40h(float)+param 03h(3d)"
          # "Solicita el contador : p.e 1240.00 Kg"
          n242 = local write "commandType"(T1."04" ("commandType")) -> ()
          n243 = Concatenate Strings(w480, w477, "0468436843" ("string"), "\r\n" ("string")) -> (w476:string)
          n244 = local write "SendString"(w476) -> ()
          n245 = call "_f_SerialComm_Hardware_Module.vi"("Command"=_f_SerialComm_Hardware_Module_Control."Write", "error in (no error)"=w497, "Write string"=w476) -> ("error out"=w494:errorcluster)  [unwired: 6 in, 2 out]
          n246 = call "Time Delay21"("error in (no error)"=w494, "Delay Time (s)"=w487) -> ("error out"=w493:errorcluster)  [unwired: 9 in]
          n247 = call "_f_SerialComm_Hardware_Module.vi"("Command"=_f_SerialComm_Hardware_Module_Control."Bytes?", "error in (no error)"=w493) -> ("error out"=w492:errorcluster, "Bytes?"=w491:u32)  [unwired: 7 in, 1 out]
          n248 = call "_f_SerialComm_Hardware_Module.vi"("Command"=_f_SerialComm_Hardware_Module_Control."Read", "error in (no error)"=w492, "Bytes to read"=w491) -> ("error out"=w485:errorcluster, "Read string"=w489:string)  [unwired: 6 in, 1 out]
          n249 = local write "ReadString"(w489) -> ()
          n250 = String Subset(string=w489, offset (0)=11, length (rest)=8 ("length (rest)")) -> (substring=w486:string)
          n251 = local write "Result"(w486) -> ()
          n252 = call "_f_IEEE754format.vi"("error in (no error)"=w485, "String"=w486) -> ("error out"=w484:errorcluster, "Number"=w482:sgl)  [unwired: 8 in]
          n253 = Number To Fractional String(number=w482, precision (6)=i16 2) -> (F-format string=w481:string)  [unwired: 2 in]
          n254 = local write "Value"(w481) -> ()
        }
        frame "WcharCounterMode" {
          # "COUNTER MODE"
          # "Command: Send/Write 01h\nProcess: 68h(104d)\nParam: 08h: 00h(char)+param 08h(8d)"
          # "0: Off\n1: Up counting\n2: Up to limit"
          n255 = To Byte Integer(number=w502) -> (8bit integer=w504:i8)
          n256 = local write "commandType"(T1."01" ("commandType")) -> ()
          n257 = Format Value(format string="%02d", value (0)=w504) -> (output string=w500:string)  [unwired: 1 in]
          n258 = Concatenate Strings(":05" ("string"), w518, "016808" ("off"), w500, "\r\n" ("string")) -> (w509:string)
          n259 = local write "SendString"(w509) -> ()
          n260 = call "_f_SerialComm_Hardware_Module.vi"("Command"=_f_SerialComm_Hardware_Module_Control."Write", "error in (no error)"=w516, "Write string"=w509) -> ("error out"=w513:errorcluster)  [unwired: 6 in, 2 out]
          n261 = call "Time Delay23"("error in (no error)"=w513, "Delay Time (s)"=w506) -> ("error out"=w512:errorcluster)  [unwired: 9 in]
          n262 = call "_f_SerialComm_Hardware_Module.vi"("Command"=_f_SerialComm_Hardware_Module_Control."Bytes?", "error in (no error)"=w512) -> ("error out"=w511:errorcluster, "Bytes?"=w510:u32)  [unwired: 7 in, 1 out]
          n263 = call "_f_SerialComm_Hardware_Module.vi"("Command"=_f_SerialComm_Hardware_Module_Control."Read", "error in (no error)"=w511, "Bytes to read"=w510) -> ("error out"=w507:errorcluster, "Read string"=w508:string)  [unwired: 6 in, 1 out]
          n264 = local write "ReadString"(w508) -> ()
        }
        frame "RcharCounterMode" {
          w525 = ":06"  # :Length
          # "Command: Request 04h\nProcess:68h(104d)\nParam: 08h: 00h(char)+param08h(8d)"
          # "Solicita el fluido actual, por si está calibrado para más de uno"
          n265 = local write "commandType"(T1."04" ("commandType")) -> ()
          n266 = Concatenate Strings(w525, w521, "0468086808" ("string"), "\r\n" ("string")) -> (w522:string)
          n267 = local write "SendString"(w522) -> ()
          n268 = call "_f_SerialComm_Hardware_Module.vi"("Command"=_f_SerialComm_Hardware_Module_Control."Write", "error in (no error)"=w538, "Write string"=w522) -> ("error out"=w535:errorcluster)  [unwired: 6 in, 2 out]
          n269 = call "Time Delay24"("error in (no error)"=w535, "Delay Time (s)"=w526) -> ("error out"=w534:errorcluster)  [unwired: 9 in]
          n270 = call "_f_SerialComm_Hardware_Module.vi"("Command"=_f_SerialComm_Hardware_Module_Control."Bytes?", "error in (no error)"=w534) -> ("error out"=w533:errorcluster, "Bytes?"=w532:u32)  [unwired: 7 in, 1 out]
          n271 = call "_f_SerialComm_Hardware_Module.vi"("Command"=_f_SerialComm_Hardware_Module_Control."Read", "error in (no error)"=w533, "Bytes to read"=w532) -> ("error out"=w529:errorcluster, "Read string"=w530:string)  [unwired: 6 in, 1 out]
          n272 = String Subset(string=w530, offset (0)=11, length (rest)=2 ("length (rest)")) -> (substring=w527:string)
          n273 = local write "ReadString"(w530) -> ()
          n274 = local write "Result"(w527) -> ()
        }
        frame "WcharCounterSPMode" {
          # "0 no setpoint change at batch limit allowed\n1 setpoint change at batch limit allowed"
          # "COUNTER SETPOINT MODE"
          # "Command: Send/Write 01h\nProcess: 68h(104d)\nParam: 05h: 00h(char)+param 05h(5d)"
          n275 = To Byte Integer(number=w543) -> (8bit integer=w545:i8)
          n276 = local write "commandType"(T1."01" ("commandType")) -> ()
          n277 = Format Value(format string="%02d", value (0)=w545) -> (output string=w541:string)  [unwired: 1 in]
          n278 = Concatenate Strings(":05" ("string"), w559, "016805" ("off"), w541, "\r\n" ("string")) -> (w550:string)
          n279 = local write "SendString"(w550) -> ()
          n280 = call "_f_SerialComm_Hardware_Module.vi"("Command"=_f_SerialComm_Hardware_Module_Control."Write", "error in (no error)"=w557, "Write string"=w550) -> ("error out"=w554:errorcluster)  [unwired: 6 in, 2 out]
          n281 = call "Time Delay26"("error in (no error)"=w554, "Delay Time (s)"=w547) -> ("error out"=w553:errorcluster)  [unwired: 9 in]
          n282 = call "_f_SerialComm_Hardware_Module.vi"("Command"=_f_SerialComm_Hardware_Module_Control."Bytes?", "error in (no error)"=w553) -> ("error out"=w552:errorcluster, "Bytes?"=w551:u32)  [unwired: 7 in, 1 out]
          n283 = call "_f_SerialComm_Hardware_Module.vi"("Command"=_f_SerialComm_Hardware_Module_Control."Read", "error in (no error)"=w552, "Bytes to read"=w551) -> ("error out"=w548:errorcluster, "Read string"=w549:string)  [unwired: 6 in, 1 out]
          n284 = local write "ReadString"(w549) -> ()
        }
        frame "RcharCounterSPMode" {
          w566 = ":06"  # :Length
          # "0 no setpoint change at batch limit allowed\n1 setpoint change at batch limit allowed"
          # "COUNTER SETPOINT MODE"
          # "Command: Send/Write 01h\nProcess: 68h(104d)\nParam: 05h: 00h(char)+param 05h(5d)"
          n285 = local write "commandType"(T1."04" ("commandType")) -> ()
          n286 = Concatenate Strings(w566, w562, "0468056805" ("string"), "\r\n" ("string")) -> (w563:string)
          n287 = local write "SendString"(w563) -> ()
          n288 = call "_f_SerialComm_Hardware_Module.vi"("Command"=_f_SerialComm_Hardware_Module_Control."Write", "error in (no error)"=w579, "Write string"=w563) -> ("error out"=w576:errorcluster)  [unwired: 6 in, 2 out]
          n289 = call "Time Delay27"("error in (no error)"=w576, "Delay Time (s)"=w567) -> ("error out"=w575:errorcluster)  [unwired: 9 in]
          n290 = call "_f_SerialComm_Hardware_Module.vi"("Command"=_f_SerialComm_Hardware_Module_Control."Bytes?", "error in (no error)"=w575) -> ("error out"=w574:errorcluster, "Bytes?"=w573:u32)  [unwired: 7 in, 1 out]
          n291 = call "_f_SerialComm_Hardware_Module.vi"("Command"=_f_SerialComm_Hardware_Module_Control."Read", "error in (no error)"=w574, "Bytes to read"=w573) -> ("error out"=w570:errorcluster, "Read string"=w571:string)  [unwired: 6 in, 1 out]
          n292 = String Subset(string=w571, offset (0)=11, length (rest)=2 ("length (rest)")) -> (substring=w568:string)
          n293 = local write "ReadString"(w571) -> ()
          n294 = local write "Result"(w568) -> ()
        }
        frame "WcharCounterNewSP" {
          # "Command: Send/Write 01h\nProcess: 68h(104d)\nParam: 06h: 00h(char)+param 06h(6d)"
          # "Envia numero entero: 0..32000"
          n295 = Multiply(x=w584, y=320.0) -> (x*y=w587:dbl)
          n296 = local write "commandType"(T1."01" ("commandType")) -> ()
          n297 = To Unsigned Word Integer(number=w587) -> (unsigned 16bit integer=w586:u16)
          n298 = Format Into String(format string="%04x", w586) -> (resulting string=w583:string)  [unwired: 2 in, 1 out]
          n299 = Concatenate Strings(":06" ("string"), w602, "016806" ("string"), w583, "\r\n" ("string")) -> (w592:string)
          n300 = local write "SendString"(w592) -> ()
          n301 = call "_f_SerialComm_Hardware_Module.vi"("Command"=_f_SerialComm_Hardware_Module_Control."Write", "error in (no error)"=w599, "Write string"=w592) -> ("error out"=w596:errorcluster)  [unwired: 6 in, 2 out]
          n302 = call "Time Delay28"("error in (no error)"=w596, "Delay Time (s)"=w582) -> ("error out"=w595:errorcluster)  [unwired: 9 in]
          n303 = call "_f_SerialComm_Hardware_Module.vi"("Command"=_f_SerialComm_Hardware_Module_Control."Bytes?", "error in (no error)"=w595) -> ("error out"=w594:errorcluster, "Bytes?"=w593:u32)  [unwired: 7 in, 1 out]
          n304 = call "_f_SerialComm_Hardware_Module.vi"("Command"=_f_SerialComm_Hardware_Module_Control."Read", "error in (no error)"=w594, "Bytes to read"=w593) -> ("error out"=w590:errorcluster, "Read string"=w591:string)  [unwired: 6 in, 1 out]
          n305 = local write "ReadString"(w591) -> ()
        }
        frame "RcharCounterNewSP" {
          w609 = ":06"  # :Length
          # "Command: Request 04h\nProcess: 68h(104d)\nParam: 06h: 00h(char)+param 06h(6d)"
          # "Solicita el numero entero (0..32000) del setpoint"
          n306 = local write "commandType"(T1."04" ("commandType")) -> ()
          n307 = Concatenate Strings(w609, w606, "0468066806" ("string"), "\r\n" ("string")) -> (w605:string)
          n308 = local write "SendString"(w605) -> ()
          n309 = call "_f_SerialComm_Hardware_Module.vi"("Command"=_f_SerialComm_Hardware_Module_Control."Write", "error in (no error)"=w622, "Write string"=w605) -> ("error out"=w619:errorcluster)  [unwired: 6 in, 2 out]
          n310 = call "Time Delay29"("error in (no error)"=w619, "Delay Time (s)"=w610) -> ("error out"=w618:errorcluster)  [unwired: 9 in]
          n311 = call "_f_SerialComm_Hardware_Module.vi"("Command"=_f_SerialComm_Hardware_Module_Control."Bytes?", "error in (no error)"=w618) -> ("error out"=w617:errorcluster, "Bytes?"=w616:u32)  [unwired: 7 in, 1 out]
          n312 = call "_f_SerialComm_Hardware_Module.vi"("Command"=_f_SerialComm_Hardware_Module_Control."Read", "error in (no error)"=w617, "Bytes to read"=w616) -> ("error out"=w615:errorcluster, "Read string"=w613:string)  [unwired: 6 in, 1 out]
          n313 = local write "ReadString"(w613) -> ()
          n314 = call "_f_BronkhorstExtract_SPPV.vi"("error in (no error)"=w615, "Read String"=w613) -> ("error out"=w614:errorcluster, "Reading"=w612:T3, "Setpoint"=w611:string)  [unwired: 7 in]
          n315 = local write "Reading"(w612) -> ()
          n316 = local write "Result"(w611) -> ()
        }
      }
      "commandType" <- T1."00" ("commandType")
    }
  }
  "error out" <- w2
